vi "adjust the waveform generator output level.vi"(10 "Amp(vpp)":dbl=1.0 format="%#_13g", 11 "Waveform Generator":refnum<visa-resource-name>) -> (3 "Waveform Generator":refnum<visa-resource-name>)   [LabVIEW 2016]
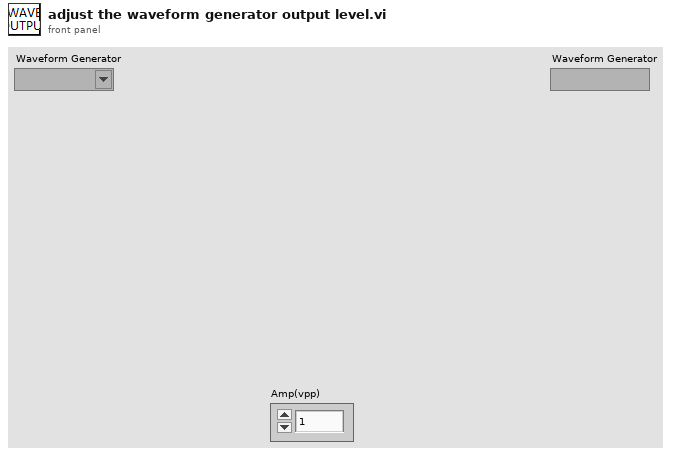
[diagram p1: front panel]
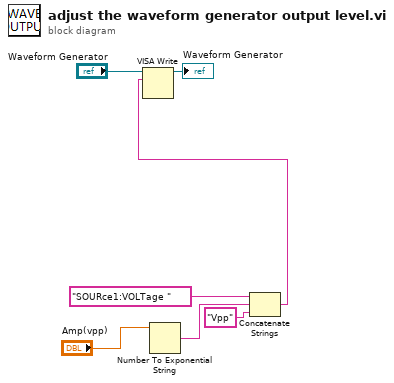
[diagram p0: block diagram]
diagram:
  n1 = Number To Exponential String(number="Amp(vpp)") -> (E-format string=w6:string)  [unwired: 3 in]
  n2 = Concatenate Strings("SOURce1:VOLTage " ("写入缓冲区"), w6, "Vpp" ("字符串")) -> (w2:string)
  n3 = VISA Write(VISA resource name="Waveform Generator", write buffer=w2) -> (VISA resource name out=→"Waveform Generator":refnum<visa-resource-name>)  [unwired: 1 in, 2 out]
